vi "DataTreeCtrl deleteFile.vi"(8 "error in (no error)":errorcluster, 11 "DataTreeCtrl in":refnum<class "DataTreeCtrl.lvclass">) -> (0 "error out":errorcluster, 3 "DataTreeCtrl out":refnum<class "DataTreeCtrl.lvclass">)   [LabVIEW 2018, in "DataTreeCtrl.lvclass"]
uses:
  DataTreeCtrl.lvclass
  DataTreeCtrl.lvclass/DataTreeCtrl.ctl
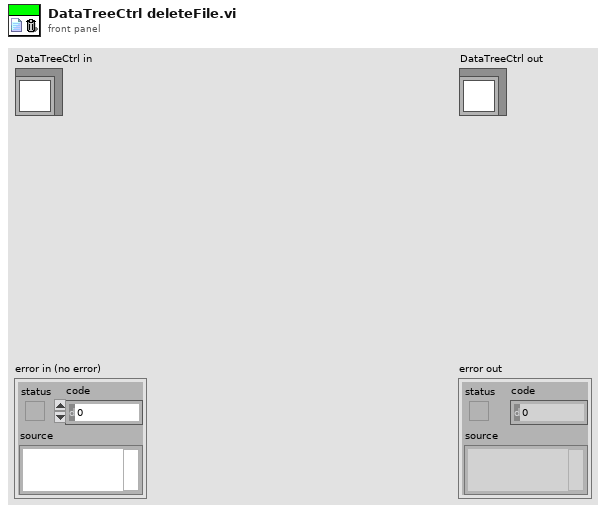
[diagram p1: front panel]
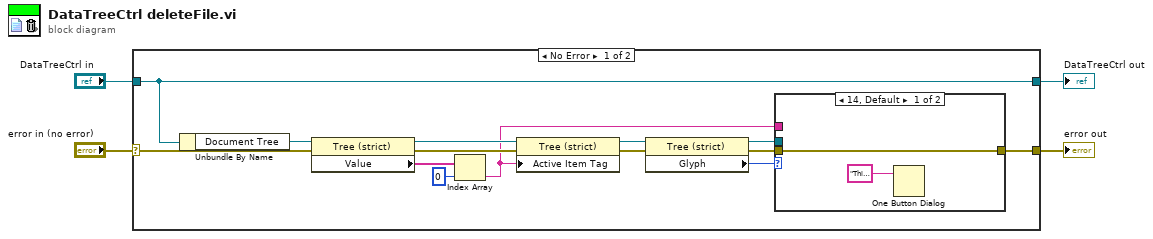
[diagram p0: block diagram]
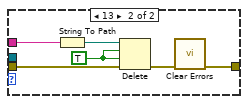
[diagram p2: hidden frame]
diagram:
  n1 = case shown="No Error" "error in (no error)" {
    selector: "error in (no error)" -> [w11 w28]
    tunnel: [w7 w28] -> w3
    tunnel: [w18 w27] -> w1
    tunnel: "DataTreeCtrl in" -> [w18 w27]
    frame No Error {
      n2 = Unbundle By Name(w18) -> ("Document Tree"=w17:refnum<vi>)
      n3 = property class="Tree (strict)"(reference=w17, error in=w11) -> (reference out=w15:refnum<vi>, error out=w12:errorcluster, "Value"=w14:string[])
      n4 = Index Array(array=w14, index=0) -> (element=w5:string)
      n5 = property class="Tree (strict)"(reference=w15, error in=w12, "Active Item Tag"=w5) -> (reference out=w10:refnum<vi>, error out=w9:errorcluster)
      n6 = property class="Tree (strict)"(reference=w10, error in=w9) -> (reference out=w6:refnum<vi>, error out=w8:errorcluster, "Glyph"=w16:i32)
      n7 = case shown="14, Default" w16 {
        tunnel: w8 -> [w19 w21]
        tunnel: [w19 w24] -> w7
        tunnel: w6 -> [_ _]
        tunnel: w5 -> [_ w23]
        frame 14, Default {
          n8 = One Button Dialog(message="This file not signal data") -> ()  [unwired: 1 in, 1 out]
        }
        frame 13 {
          w26 = TRUE ("confirm (F)")
          n9 = String To Path(string=w23) -> (path=w22:path)
          n10 = Delete(path (use dialog)=w22, entire hierarchy (F)=w26, confirm (F)=w26, error in=w21) -> (error out=w25:errorcluster)  [unwired: 1 in, 2 out]
          n11 = call <vilib>:"Clear Errors.vi"("error in (no error)"=w25) -> ("error out"=w24:errorcluster)  [unwired: 5 in, 1 out]
        }
      }
    }
    frame Error {
    }
  }
  "error out" <- w3
  "DataTreeCtrl out" <- w1
